vi "HFRR ADV v01.vi"() -> ()   [LabVIEW 2025] (continued)
              }
            }
          }
          frame Enabled {
          }
        }
        n3589 = local read "Quit"() -> (w4325:bool)
      }
    }
    frame Enabled {
    }
  }
  n3590 = stacked-sequence {
    tunnel: [w4723] -> w35
    frame #0 {
      w4723 = FALSE ("Upload \nConfirmed")
      n3591 = local write "Upload \nConfirmed"(w4723) -> ()
      n3592 = local write "St Str"("") -> ()
    }
  }
  n3593 = disable-structure shown="Disabled" {
    disable-tunnel: w35 -> [w4724 _]
    frame Disabled {
      n3594 = case shown="True" {
        selector: _ -> [_ _]
        tunnel: w4724 -> [_ w4725]
        frame False {
        }
        frame True {
          n3595 = while {
            tunnel: [w4731] -> _
            tunnel: w4725 -> [_]
            i -> [w4731]
            stop <- w4726 stop-if-true
            n3596 = local read "Json End Flg"() -> (w4730:bool)
            n3597 = Wait (ms)(milliseconds to wait=u32 20 ("Refresh Rate (ms)")) -> ()  [unwired: 1 out]
            n3598 = local read "refresh flag"() -> (w4727:bool)
            n3599 = local read "RUN"() -> (w4728:bool)
            n3600 = And(x=w4728, y=w4727) -> (x .and. y?=w4729:bool)
            n3601 = Or(x=w4729, y=w4730) -> (x .or. y?=w4732:bool)
            "AR Led" <- w4732
            n3602 = case shown="True" w4732 {
              frame False {
              }
              frame True {
                w4749 = "\",\""
                n3603 = local read "UUID"() -> (w4747:string)
                n3604 = local write "refresh flag"(FALSE ("refresh flag")) -> ()
                n3605 = local read "time"() -> (w4736:dbl)
                n3606 = Multiply(x=w4736, y=60.0) -> (x*y=w4735:dbl)
                n3607 = Concatenate Strings("UUID\" : \"", w4747, "\"}") -> (w4750:string)
                n3608 = Number To Fractional String(number=w4735, width (-)=i16 10, precision (6)=i16 4) -> (F-format string=w4764:string)  [unwired: 1 in]
                n3609 = Concatenate Strings("{", "\"Time\":\"", w4764, w4749) -> (w4759:string)
                n3610 = stacked-sequence {
                  tunnel: w4749 -> [w4812 w4820 w4827 w4835 w4843 w4852 w4859]
                  tunnel: [w4813 _ _ _ _ _ _] -> w4763
                  tunnel: [_ w4821 _ _ _ _ _] -> w4762
                  tunnel: [_ _ w4828 _ _ _ _] -> w4761
                  tunnel: [_ _ _ w4837 _ _ _] -> w4760
                  tunnel: w4750 -> [_ _ _ _ _ _ w4870]
                  tunnel: [_ _ _ _ _ _ w4869] -> w4746
                  tunnel: [_ _ _ _ _ w4849 _] -> w4745
                  tunnel: [_ _ _ _ w4842 _ _] -> w4744
                  frame #0 {
                    n3611 = local read "NORMAL LOAD"() -> (w4811:dbl)
                    n3612 = Number To Fractional String(number=w4811, width (-)=i16 10, precision (6)=i16 4) -> (F-format string=w4814:string)  [unwired: 1 in]
                    n3613 = Concatenate Strings("NormalLoad\":\"", w4814, w4812) -> (w4813:string)
                  }
                  frame #1 {
                    n3614 = local read "Temp"() -> (w4819:dbl)
                    n3615 = Number To Fractional String(number=w4819, width (-)=i16 10, precision (6)=i16 4) -> (F-format string=w4822:string)  [unwired: 1 in]
                    n3616 = Concatenate Strings("Temperature\":\"", w4822, w4820) -> (w4821:string)
                  }
                  frame #2 {
                    n3617 = local read "cof"() -> (w4825:dbl)
                    n3618 = Number To Fractional String(number=w4825, width (-)=i16 10, precision (6)=i16 4) -> (F-format string=w4829:string)  [unwired: 1 in]
                    n3619 = Concatenate Strings("FrictionalForce\":\"", w4829, w4827) -> (w4828:string)
                  }
                  frame #3 {
                    n3620 = local read "Set Hz"() -> (w4833:dbl)
                    n3621 = Multiply(x=w4833, y=60.0) -> (x*y=w4832:dbl)
                    n3622 = Number To Fractional String(number=w4832, width (-)=i16 10, precision (6)=i16 4) -> (F-format string=w4838:string)  [unwired: 1 in]
                    n3623 = Concatenate Strings("Speed\":\"", w4838, w4835) -> (w4837:string)
                  }
                  frame #4 {
                    n3624 = local read item#-1() -> (w4841)
                    n3625 = Number To Fractional String(number=w4841, width (-)=i16 10, precision (6)=i16 4) -> (F-format string=w4845:string)  [unwired: 1 in]
                    n3626 = Concatenate Strings("LinearDeformation\":\"", w4845, w4843) -> (w4842:string)
                  }
                  frame #5 {
                    n3627 = local read "AIR TEMP"() -> (w4848:dbl)
                    n3628 = local read "Json St Flg"() -> (w4850:bool)
                    n3629 = local read "Json End Flg"() -> (w4851:bool)
                    n3630 = Number To Fractional String(number=w4848, width (-)=i16 10, precision (6)=i16 4) -> (F-format string=w4854:string)  [unwired: 1 in]
                    n3631 = Concatenate Strings("Vibration\":\"", w4854, w4852) -> (w4849:string)
                    n3632 = And(x=w4850, y=w4851) -> ()  [unwired: 1 out]
                  }
                  frame #6 {
                    n3633 = local read "Json End Flg"() -> (w4858:bool)
                    n3634 = Get Date/Time In Seconds() -> (seconds since 1Jan1904=w4866:timestamp)
                    n3635 = local read "Json St Flg"() -> (w4857:bool)
                    n3636 = To Double Precision Float(number=w4866) -> (double precision float=w4865:dbl)
                    n3637 = Subtract(x=w4865, y=2082844800.0) -> (x-y=w4863:dbl)
                    n3638 = Number To Fractional String(number=w4863, width (-)=i16 12, precision (6)=i16 0) -> (F-format string=w4860:string)  [unwired: 1 in]
                    n3639 = case shown="True" w4858 {
                      tunnel: ["" w4873] -> w4867
                      tunnel: w4860 -> [_ w4874]
                      tunnel: w4859 -> [_ w4872]
                      frame False {
                      }
                      frame True {
                        n3640 = local write "Json End Flg"(FALSE ("Json St Flg")) -> ()
                        n3641 = Concatenate Strings("End\": \"", w4874, w4872) -> (w4873:string)
                      }
                    }
                    n3642 = case shown="True" w4857 {
                      tunnel: [w4877 w4880] -> w4868
                      tunnel: w4860 -> [_ w4881]
                      tunnel: w4859 -> [_ w4878]
                      frame False {
                        n3643 = local read "St Str"() -> (w4877:string)
                      }
                      frame True {
                        n3644 = Concatenate Strings("Start\":\"", w4881, w4878) -> (w4880:string)
                        "St Str" <- w4880
                        n3645 = local write "Json St Flg"(FALSE ("Json St Flg")) -> ()
                      }
                    }
                    n3646 = Concatenate Strings(w4868, w4867, w4870) -> (w4869:string)
                  }
                }
                n3647 = local read "FILE"() -> (w4738:string)
                n3648 = Concatenate Strings("\",\"OperatorID\":\"" ("string"), "Operator ID") -> (w4741:string)
                n3649 = Concatenate Strings("\",\"DatasetTitle\":\"" ("string"), w4738) -> (w4740:string)
                n3650 = Concatenate Strings("\",\"SerialNumber\":\"" ("string"), "Serial No") -> (w4770:string)
                n3651 = Concatenate Strings("\",\"ModelNumber\":\"" ("string"), "Model No") -> (w4769:string)
                n3652 = Concatenate Strings(w4770, w4769) -> (w4752:string)
                n3653 = Concatenate Strings("{\"SecretKey\":\"", "Secret Key", w4752, w4741, w4740, "\",\"Samples\":[") -> (w4757:string)
                n3654 = Concatenate Strings(w4759, w4763, w4762, w4761, w4760, w4744, w4745, w4746) -> (w4758:string)
                n3655 = Concatenate Strings(w4757, w4758, "]}") -> (w4756:string)
                n3656 = stacked-sequence {
                  tunnel: w4756 -> [w4785 _ _]
                  tunnel: [_ _ w4802] -> _
                  frame #0 {
                    (unwired) FALSE ("convert eol (F)")
                    w4787 = enum16{"start", "end", "current"}."start" ("pos mode (0:2)")
                    n3657 = Path To String(path="Path") -> (string=w4793:string)
                    n3658 = Concatenate Strings(w4793, "\\", "Data File Name") -> (w4795:string)
                    n3659 = local write "standard output"(" ") -> ()
                    n3660 = String To Path(string=w4795) -> (path=w4784:path)
                    n3661 = call <vilib>:"Open_Create_Replace File.vi"("advisory dialog? (display:T)"=FALSE, "function (open:0)"=T27."create or replace", "file path"=w4784) -> ("error out"=w4798:errorcluster, "refnum"=w4797:refnum<file>)  [unwired: 5 in, 2 out]
                    n3662 = Set File Position(refnum=w4797, from (0:start)=w4787, error in=w4798) -> (refnum out=w4778:refnum<file>, error out=w4777:errorcluster)  [unwired: 1 in]
                    n3663 = Write to Binary File(file (use dialog)=w4778, data=" ", error in=w4777, 5:FALSE ("prepend array or string size? (T)")) -> (refnum out=w4788:refnum<file>, error out=w4789:errorcluster)  [unwired: 2 in, 1 out]
                    n3664 = Set File Position(offset (in bytes) (0)=w4787, refnum=w4788, error in=w4789) -> (refnum out=w4781:refnum<file>, error out=w4780:errorcluster)  [unwired: 1 in]
                    n3665 = Write to Binary File(file (use dialog)=w4781, data=w4785, error in=w4780, 5:FALSE ("prepend array or string size? (T)")) -> (error out=w4783:errorcluster)  [unwired: 2 in, 2 out]
                    n3666 = flat-sequence {
                      tunnel: w4784 -> [w4800]
                      tunnel: w4783 -> [_]
                      frame #0 {
                        n3667 = call <vilib>:"Read Characters From File.vi"("file path (dialog if empty)"=w4800) -> ("character string"=→"JSON string":string)  [unwired: 5 in, 3 out]
                      }
                    }
                    "SinglePoint" <- w4785
                  }
                  frame #1 {
                  }
                  frame #2 {
                    (unwired) "\"Stored\": true" ("string")
                    n3668 = call <vilib>:"System Exec.vi"("run minimized? (F)"=TRUE, "wait until completion? (T)"=TRUE, "working directory"=path "C:/LAB-IQ-NXT", "command line"="C:\\LAB-IQ-NXT\\JPost.bat") -> ("standard error"=→"Respose From Server":string, "standard output"=w4805:string)  [unwired: 4 in, 2 out]
                    "standard output" <- w4805
                    n3669 = Match Pattern(string=w4805, regular expression="JSON Check String") -> (match substring=w4803:string, offset past match=w4802:i32)  [unwired: 1 in, 2 out]
                    n3670 = Equal?(x=w4803, y="JSON Check String") -> (x = y?=→"Upload \nConfirmed":bool)
                  }
                }
              }
            }
            n3671 = local read "Quit"() -> (w4726:bool)
          }
        }
      }
    }
    frame Enabled {
    }
  }
  n3672 = disable-structure shown="Disabled" {
    disable-tunnel: _ -> [w4888 _]
    frame Disabled {
      n3673 = while {
        shift-right: [w4896] -> w4884
        shift-left: _ -> [w4897]
        shift-right: [w4894] -> w4885
        shift-left: errorcluster {"status"=TRUE, "code"=0, "source"="Init"} ("error out") -> [w4895]
        shift-right: [w4892] -> _
        shift-left: "" -> [w4893]
        tunnel: [w4890] -> _
        tunnel: w4888 -> [_]
        i -> [w4890]
        stop <- w4889 stop-if-true
        n3674 = flat-sequence {
          tunnel: [w4898] -> w4891
          frame #0 {
            n3675 = Wait (ms)(milliseconds to wait=10.0 ("Delay")) -> (millisecond timer value=w4898:u32)
          }
        }
        n3676 = case shown="No Error" w4895 {
          selector: w4895 -> [w4931 w5053]
          tunnel: [w4913 w5055] -> w4896
          tunnel: [w4912 w5054] -> w4894
          tunnel: w4897 -> [w4932 w5047]
          tunnel: w4893 -> [w4911 w5046]
          tunnel: [w4910 w5046] -> w4892
          tunnel: w4891 -> [_ _]
          frame No Error {
            n3677 = Concatenate Strings("COMMAND", "\r", "\n") -> (w4922:string)
            n3678 = case shown="True" "Measure" {
              tunnel: w4932 -> [w4958 w4965]
              tunnel: w4931 -> [w4957 w4964]
              tunnel: [w4958 w4963] -> w4930
              tunnel: [w4957 w4962] -> w4909
              tunnel: w4922 -> [_ w4961]
              frame False {
              }
              frame True {
                n3679 = VISA Write(VISA resource name=w4965, write buffer=w4961, error in (no error)=w4964) -> (VISA resource name out=w4963:refnum<visa-resource-name>, error out=w4962:errorcluster)  [unwired: 1 out]
                n3680 = local write "Read String"("") -> ()
                n3681 = local write "Measure"(FALSE) -> ()
              }
            }
            n3682 = property class="Instr"(reference=w4930, error in=w4909) -> (reference out=w4929:refnum<visa-resource-name>, error out=w4928:errorcluster, "Serial Settings:Number of Bytes at Serial Port"=w4927:u32)
            n3683 = Greater?(x=w4927, y=u32 100) -> (0:w4925:bool)
            n3684 = case shown="True" w4925 {
              tunnel: w4929 -> [w4968 w4993]
              tunnel: w4928 -> [w4967 w4992]
              tunnel: w4927 -> [_ w4991]
              tunnel: [w4968 w4990] -> w4915
              tunnel: [w4967 w4989] -> w4914
              tunnel: w4911 -> [w4966 w4988]
              tunnel: [w4966 ""] -> w4910
              frame False {
              }
              frame True {
                w4978 = u32 6 ("y")
                # "Page 84 of \nmanual"
                n3685 = VISA Read(VISA resource name=w4993, byte count=w4991, error in (no error)=w4992) -> (VISA resource name out=w4990:refnum<visa-resource-name>, read buffer=w4986:string, error out=w4989:errorcluster)  [unwired: 1 out]
                n3686 = while {
                  tunnel: w4986 -> [w5042]
                  tunnel: [w5038] -> w4980 mode=indexing
                  tunnel: [w5032] -> w4984 mode=indexing
                  tunnel: [w5030] -> _
                  i -> [w5030]
                  stop <- w5035 stop-if-true
                  n3687 = String Subset(string=w5042, offset (0)=w5030) -> (substring=w5037:string)  [unwired: 1 in]
                  n3688 = String To Byte Array(string=w5037) -> (unsigned byte array=w5041:u8[])
                  n3689 = String Length(string=w5037) -> (length=w5036:i32)
                  n3690 = Index Array(array=w5041) -> (element=w5040:u8)  [unwired: 1 in]
                  n3691 = Equal To 0?(x=w5036) -> (x = 0?=w5035:bool)
                  n3692 = Number To Boolean Array(number=w5040) -> (Boolean array=w5034:bool[])
                  n3693 = Reverse 1D Array(array=w5034) -> (reversed array=w5033:bool[])
                  n3694 = And(x=w5034, y=bool[] [FALSE, FALSE, FALSE, FALSE, FALSE, FALSE, TRUE, TRUE] ("Boolean array")) -> (x .and. y?=w5038:bool[])
                  n3695 = And(x=w5033, y=bool[] [FALSE, FALSE, TRUE, TRUE, TRUE, TRUE, TRUE, TRUE] ("Boolean array")) -> (x .and. y?=w5032:bool[])
                }
                n3696 = Concatenate Strings(w4988, w4986) -> (→"Read String":string)
                n3697 = while {
                  tunnel: w4980 -> [w5029] mode=indexing
                  tunnel: [w5025] -> w4983
                  i -> [w5025]
                  stop <- w5026 stop-if-true
                  n3698 = Search 1D Array(1D array=w5029, element=TRUE) -> (index of element=w5027:i32)  [unwired: 1 in]
                  n3699 = Less Than 0?(x=w5027) -> (x < 0?=w5026:bool)
                }
                n3700 = Delete From Array(array=w4984, length=w4983, index (row)=0) -> (array with subset deleted=w4979:bool[][])  [unwired: 1 in, 1 out]
                n3701 = Array Size(array=w4979) -> (size(s)=w4981:i32[])
                n3702 = Index Array(array=w4981) -> (element=w4973:i32)  [unwired: 1 in]
                n3703 = Greater?(x=w4973, y=w4978) -> (0:w4976:bool)
                n3704 = Subtract(x=w4973, y=w4978) -> (x-y=w4977:u32)
                n3705 = Select(t=w4977, s=w4976, f=u32 0) -> (s? t:f=w4974:u32)
                n3706 = while {
                  tunnel: w4979 -> [w5012]
                  tunnel: [w5014] -> w4972 mode=indexing
                  tunnel: w4974 -> [w4996]
                  i -> [w5013]
                  stop <- w5011 stop-if-true
                  w5003 = 6 ("index")
                  w5002 = 2 ("length")
                  # "Page 65 of \nmanual"
                  n3707 = Multiply(x=u32 3 ("y"), y=w5013) -> (x*y=w5010:u32)
                  n3708 = Divide(x=u32 102 ("y"), y=u32 65520) -> (x/y=w5020:dbl)
                  n3709 = Greater Or Equal?(x=w5010, y=w4996) -> (x >= y?=w5011:bool)
                  n3710 = Index Array(array=w5012, index (row) #1=w5010) -> (element #1=w5008:bool[], element #2=w5007:bool[], element #3=w5006:bool[])  [unwired: 5 in]
                  n3711 = Reverse 1D Array(array=w5008) -> (reversed array=w5001:bool[])
                  n3712 = Reverse 1D Array(array=w5007) -> (reversed array=w5005:bool[])
                  n3713 = Reverse 1D Array(array=w5006) -> (reversed array=w5004:bool[])
                  n3714 = Delete From Array(array=w5001, length=w5002, index=w5003) -> (array with subset deleted=w4997:bool[])  [unwired: 1 out]
                  n3715 = Delete From Array(array=w5005, length=w5002, index=w5003) -> (array with subset deleted=w4998:bool[])  [unwired: 1 out]
                  n3716 = Delete From Array(array=w5004, length=w5002, index=w5003) -> (array with subset deleted=w4999:bool[])  [unwired: 1 out]
                  n3717 = Insert Into Array(array=bool[] [] ("Boolean array"), new element #1=w4997, new element #2=w4998, new element #3=w4999) -> (w5000:bool[])  [unwired: 1 in]
                  n3718 = Boolean Array To Number(Boolean array=w5000) -> (number=w5009:u32)
                  n3719 = Multiply(x=w5020, y=w5009) -> (x*y=w5019:dbl)
                  n3720 = Decrement(x=w5019) -> (x-1=w5018:dbl)
                  n3721 = Divide(x=w5018, y=u32 100) -> (x/y=w5016:dbl)
                  n3722 = Multiply(x=w5016, y=u32 10) -> (x*y=w5014:dbl)
                }
                n3723 = Delete From Array(array=w4972) -> (array with subset deleted=w4971:dbl[])  [unwired: 2 in, 1 out]
                "Waveform Graph 5" <- w4971
                "Waveform Chart 3" <- w4971
                n3724 = call-poly <vilib>:"Mean.vi"("X"=w4971) -> ("mean"=w4970:dbl)  [unwired: 1 out]
                "Measure_LDS" <- w4970
                n3725 = case shown="True" "Zero 4" {
                  tunnel: w4970 -> [_ w4995]
                  frame False {
                  }
                  frame True {
                    n3726 = local write "Zero 4"(FALSE ("Zero 4")) -> ()
                    "z_measure" <- w4995
                  }
                }
              }
            }
            n3727 = local read "Measure_LDS"() -> (w4905:dbl)
            n3728 = local read "Boolean 7"() -> (w4903:bool)
            n3729 = local read "Boolean 8"() -> (w4902:bool)
            n3730 = local read item#-1() -> (w4904)
            n3731 = case shown="True" "Boolean 8" {
              tunnel: w4904 -> [_ w4935]
              tunnel: w4905 -> [_ w4934]
              frame False {
              }
              frame True {
                n3732 = local read "Captured Values 2"() -> (w4938:dbl[][])
                n3733 = Build Array(w4935, w4934) -> (w4933:dbl[])
                n3734 = Build Array (concatenate)(w4938, w4933) -> (w4936:dbl[][])
                n3735 = local write "Captured Values 2"(w4936) -> ()
                n3736 = local write "Boolean 8"(FALSE ("Boolean 8")) -> ()
              }
            }
            n3737 = call "Build XY Graph"("Enable"=w4902, "Reset"=w4903, "Y Input"=w4905, "X Input"=w4904) -> ("XY Graph"=→"?":cluster{"Y":dbl[], "Y":dbl[]}[])  [unwired: 6 in, 1 out]
            n3738 = case shown="True" "Boolean 9" {
              frame False {
              }
              frame True {
                n3739 = local read "Captured Values 2"() -> (w4940:dbl[][])
                n3740 = Index Array(array=w4940, index (col) #1=0 ("disabled index (col)"), index (col) #2=1 ("index (col)")) -> (element #1=w4943:dbl[], element #2=w4942:dbl[])  [unwired: 2 in]
                n3741 = call <vilib>:"Linear Fit.vi"("Y"=w4943, "X"=w4942) -> ("slope"=→"Slope":dbl, "intercept"=→"Intercept":dbl)  [unwired: 9 in, 3 out]
                n3742 = local write "Boolean 9"(FALSE ("Boolean 9")) -> ()
              }
            }
            n3743 = case shown="True" "Boolean 7" {
              frame False {
              }
              frame True {
                n3744 = local write "Captured Values 2"(dbl[][] [] ("Captured Values")) -> ()
                n3745 = local write "Boolean 7"(FALSE ("Boolean 7")) -> ()
              }
            }
            n3746 = Concatenate Strings("COMMAND 2", "\r", "\n") -> (w4917:string)
            n3747 = case shown="True" "Measure 2" {
              tunnel: w4915 -> [w4950 w4956]
              tunnel: w4914 -> [w4949 w4955]
              tunnel: [w4950 w4954] -> w4913
              tunnel: [w4949 w4953] -> w4912
              tunnel: w4917 -> [_ w4952]
              frame False {
              }
              frame True {
                n3748 = local write "Measure 2"(FALSE ("WRITE")) -> ()
                n3749 = VISA Write(VISA resource name=w4956, write buffer=w4952, error in (no error)=w4955) -> (VISA resource name out=w4954:refnum<visa-resource-name>, error out=w4953:errorcluster)  [unwired: 1 out]
              }
            }
          }
          frame Error {
            w5045 = u16 10 items=["1.0"=10, "1.5"=15, "2.0"=20] ("stop bits (10: 1 bit)")
            n3750 = Wait (ms)(milliseconds to wait=u32 20) -> ()  [unwired: 1 out]
            n3751 = VISA Close(VISA resource name=w5047, error in (no error)=w5053) -> (error out=w5052:errorcluster)
            n3752 = call <vilib>:"Clear Errors.vi"("error in (no error)"=w5052) -> ("error out"=w5051:errorcluster)  [unwired: 5 in, 1 out]
            n3753 = call-poly "VISA Configure Serial Port"("VISA resource name"="Laser Disp Sensor", "timeout (10sec)"=u32 200, "Enable Termination\nChar (T)"=TRUE ("Enable Termination\nChar (T)"), "baud rate (9600)"=u32 921600, "error in (no error)"=w5051, "stop bits (10: 1 bit)"=w5045) -> ("VISA resource name out"=w5055:refnum<visa-resource-name>, "error out"=w5054:errorcluster)  [unwired: 8 in]
          }
        }
        n3754 = local read "Quit"() -> (w4889:bool)
      }
      n3755 = VISA Close(VISA resource name=w4884, error in (no error)=w4885) -> (error out=w4883:errorcluster)
      n3756 = call <vilib>:"Clear Errors.vi"("error in (no error)"=w4883) -> ()  [unwired: 5 in, 2 out]
    }
    frame Enabled {
    }
  }
  n3757 = disable-structure shown="Disabled" {
    disable-tunnel: _ -> [w5060 _]
    frame Disabled {
      n3758 = while {
        tunnel: [w5067] -> _
        shift-right: [w5064] -> w5057
        shift-left: _ -> [w5066]
        shift-right: [w5065] -> w5058
        shift-left: errorcluster {"status"=TRUE, "code"=0, "source"="Init"} ("error out") -> [w5063]
        tunnel: w5060 -> [_]
        i -> [w5067]
        stop <- w5061 stop-if-true
        n3759 = flat-sequence {
          tunnel: w5063 -> [w5158]
          tunnel: [w5158] -> w5062
          frame #0 {
            n3760 = Wait (ms)(milliseconds to wait=u32 50) -> ()  [unwired: 1 out]
          }
        }
        n3761 = case shown="No Error" w5062 {
          selector: w5062 -> [w5108 w5151]
          tunnel: w5066 -> [w5107 w5150]
          tunnel: [w5074 w5141] -> w5065
          tunnel: [w5075 w5149] -> w5064
          frame No Error {
            w5101 = T28 {"Mode"=enum."RTU", "Slave Address"=1} ("Serial Parameters")
            n3762 = call-poly <vilib>:"MB Serial Master Query (poly).vi"("VISA resource name"=w5107, "Starting Address"=i16 1000, "Quantity"=u16 1, "Timeout"=u32 1000, "error in"=w5108, "Serial Parameters"=w5101) -> ("VISA resource name out"=w5102:refnum<visa-resource-name>, "Input Registers"=w5104:u16[], "error out"=w5100:errorcluster)  [unwired: 10 in, 1 out]
            n3763 = Random Number (0-1)() -> (number: 0 to 1=w5089:dbl)
            n3764 = Index Array(array=w5104, index=0) -> (element=w5099:u16)
            n3765 = Subtract(x=w5089, y=0.5) -> (x-y=w5088:dbl)
            n3766 = Divide(x=w5099, y=10 ("index")) -> (x/y=w5093:dbl)
            n3767 = Multiply(x=w5088, y=0.5) -> (x*y=w5087:dbl)
            n3768 = Add(x=w5093, y=w5087) -> (x+y=w5092:dbl)
            n3769 = local read "Amb temp"() -> (w5076:dbl)
            n3770 = Multiply(x=w5092, y=0.2) -> (x*y=w5096:dbl)
            n3771 = Multiply(x=w5076, y=0.8) -> (x*y=w5094:dbl)
            n3772 = Add(x=w5096, y=w5094) -> (x+y=w5077:dbl)
            n3773 = local read "set temp old"() -> (w5071:dbl)
            n3774 = local write "Amb temp"(w5077) -> ()
            n3775 = Select(t="SetTemp 2", s="Heater", f=100.0) -> (s? t:f=w5072:dbl)
            n3776 = Not Equal?(x=w5072, y=w5071) -> (x != y?=w5070:bool)
            n3777 = case shown="True" w5070 {
              tunnel: w5102 -> [w5136 w5138]
              tunnel: [w5135 w5138] -> w5082
              tunnel: w5100 -> [w5134 w5137]
              tunnel: [w5133 w5137] -> w5080
              tunnel: w5072 -> [w5128 _]
              tunnel: w5101 -> [w5130 w5139]
              tunnel: [w5130 w5139] -> w5083
              frame True {
                n3778 = Multiply(x=w5128, y=10 ("index")) -> (x*y=w5127:dbl)
                n3779 = call-poly <vilib>:"MB Serial Master Query (poly).vi"("VISA resource name"=w5136, "Address"=u16 0, "Holding Register"=w5127, "Timeout"=u32 1000, "error in"=w5134, "Serial Parameters"=w5130) -> ("VISA resource name out"=w5135:refnum<visa-resource-name>, "error out"=w5133:errorcluster)  [unwired: 11 in, 1 out]
                "set temp old" <- w5128
              }
              frame False {
              }
            }
            n3780 = flat-sequence {
              tunnel: [w5109] -> _
              tunnel: [w5109] -> w5079
              tunnel: w5080 -> [w5109]
              frame #0 {
                n3781 = Wait (ms)(milliseconds to wait=u32 100) -> ()  [unwired: 1 out]
              }
            }
            n3782 = call "Elapsed Time12"("Time Target (s)"=2.0, "Auto Reset"=TRUE) -> ("Time has Elapsed"=w5084:bool)  [unwired: 10 in, 7 out]
            n3783 = case shown="True" w5084 {
              tunnel: w5083 -> [w5113 w5126]
              tunnel: [w5113 w5126] -> _
              tunnel: [w5112 w5124] -> w5075
              tunnel: w5082 -> [w5112 w5125]
              tunnel: [w5111 w5122] -> w5074
              tunnel: w5079 -> [w5111 w5123]
              frame False {
              }
              frame True {
                n3784 = call-poly <vilib>:"MB Serial Master Query (poly).vi"("VISA resource name"=w5125, "Starting Address"=i16 1003 ("Addr"), "Quantity"=u16 1, "Timeout"=u32 1000, "error in"=w5123, "Serial Parameters"=w5126) -> ("VISA resource name out"=w5124:refnum<visa-resource-name>, "Input Registers"=w5119:u16[], "error out"=w5122:errorcluster)  [unwired: 10 in, 1 out]
                n3785 = Index Array(array=w5119, index=0) -> (element=w5118:u16)
                n3786 = Divide(x=w5118, y=u16 10) -> (x/y=w5114:dbl)
                n3787 = local write "set temp old"(w5114) -> ()
                n3788 = local write "SetTemp"(w5114) -> ()
              }
            }
            "Error Code" <- w5074
            n3789 = Unbundle(w5074) -> ("status"=→"TK4 status":bool)  [unwired: 2 out]
            "SetTemp" <- "SetTemp 2"
          }
          frame Error {
            w5153 = u16 0 items=["None", "Odd", "Even", "Mark", "Space"] ("Parity")
            w5154 = u16 0 items=["None", "XON/XOFF", "RTS/CTS", "XON/XOFF & RTS/CTS", "DTR/DSR", "XON/XOFF & DTR/DSR"] ("Flow Control")
            n3790 = VISA Clear(VISA resource name=w5150, error in (no error)=w5151) -> (VISA resource name out=w5144:refnum<visa-resource-name>, error out=w5142:errorcluster)
            n3791 = VISA Close(VISA resource name=w5144, error in (no error)=w5142) -> (error out=w5143:errorcluster)
            n3792 = call <vilib>:"Clear Errors.vi"("error in (no error)"=w5143) -> ("error out"=w5152:errorcluster)  [unwired: 5 in, 1 out]
            n3793 = Unbundle By Name(T28 {"Mode"=enum."RTU", "Slave Address"=1} ("input cluster")) -> ("Mode"=w5155:enum16{"RTU", "ASCII"})
            n3794 = call <vilib>:"MB Serial Init.vi"("Timeout"=u32 100, "Flow Control"=w5154, "Mode"=w5155, "error in (no error)"=w5152, "Parity"=w5153, "Baud Rate"=u32 9600, "VISA resource name"="Lubrication System COM Port :") -> ("error out"=w5141:errorcluster, "VISA resource name out"=w5149:refnum<visa-resource-name>)  [unwired: 3 in]
            n3795 = local write "set temp old"(0.0 ("set temp old")) -> ()
            n3796 = Unbundle(w5141) -> ("status"=w5140:bool)  [unwired: 2 out]
            n3797 = case shown="True" w5140 {
              selector: w5140 -> [_ w5157]
              frame False {
              }
              frame True {
                n3798 = local write "TK4 status"(w5157) -> ()
              }
            }
          }
        }
        n3799 = local read "Quit"() -> (w5061:bool)
      }
      n3800 = VISA Close(VISA resource name=w5057, error in (no error)=w5058) -> (error out=w5056:errorcluster)
      n3801 = call <vilib>:"Clear Errors.vi"("error in (no error)"=w5056) -> ()  [unwired: 5 in, 2 out]
    }
    frame Enabled {
    }
  }
